vi "Set State.vi"(0 "Controller in":refnum<class "Controller.lvclass">, 1 "State":bool, 5 "error in":errorcluster) -> (14 "Controller out":refnum<class "Controller.lvclass">, 19 "error out":errorcluster)   [LabVIEW 2014, in "Controller.lvlib" / "Change Filter State.lvclass"]
uses:
  Change Filter State.lvclass
  Controller.lvclass
  SuperActor/Ex Nested.lvclass/Ex Nested.ctl
  Controller.lvclass/Controller.ctl
  <vilib>/DAQmx/write.llb/DAQmx Write (Digital 1D Bool NChan 1Samp 1Line).vi
  SuperActor/Read CVT Session.vi
  SuperActor/Read Log Session.vi
  Accessors/Read Filter Task.vi
  Accessors/Read Switch DVR.vi
  <vilib>/DAQmx/miscellaneous.llb/DAQmx Fill In Error Info.vi
  <userlib>/_Session Fwk/Session - Root.lvclass
  reusable/Switch/Switch.lvclass
  reusable/Session APIs/Session Log/System Log.lvclass
  reusable/Session APIs/CVT/CVT.lvclass
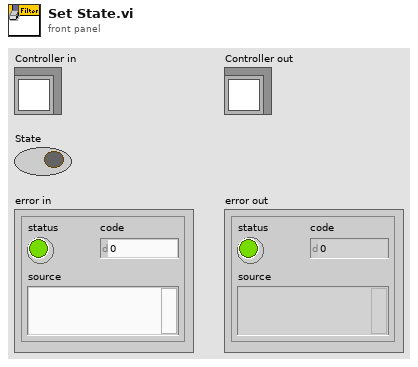
[diagram p1: front panel]
types:
  T1 = typedef "Session - Root.lvclass/Session Handle.ctl" = refnum<data-value>
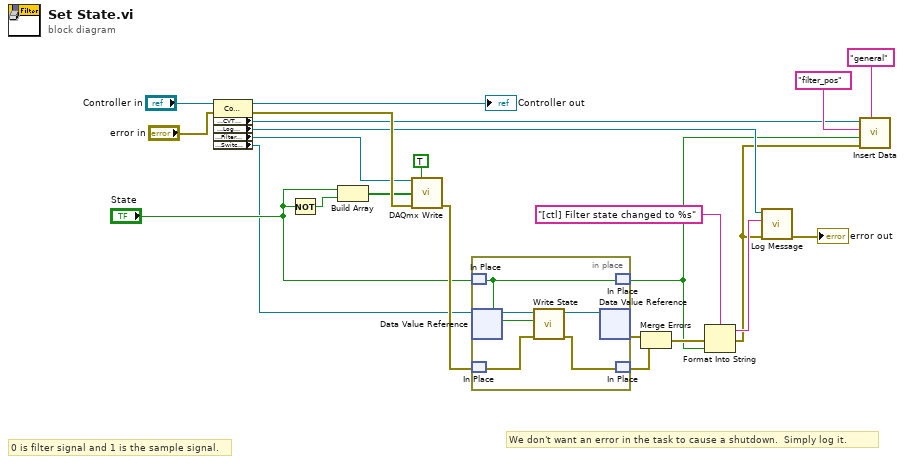
[diagram p0: block diagram]
diagram:
  # "0 is filter signal and 1 is the sample signal."
  # "We don't want an error in the task to cause a shutdown.  Simply log it."
  n1 = property class="Controller"(reference="Controller in", error in="error in") -> (reference out=→"Controller out":refnum<class "Controller.lvclass">, error out=w17:errorcluster, "Accessors:CVT Session"=w10:T1, "Accessors:Log Session"=w11:T1, "Accessors:Filter Task"=w1:refnum<k21>, "Accessors:Switch DVR"=w2:refnum<data-value>)
  n2 = Not(x="State") -> (.not. x?=w16:bool)
  n3 = Build Array("State", w16) -> (w15:bool[])
  n4 = call-poly <vilib>:"DAQmx Write.vi"("task/channels in"=w1, "auto start"=TRUE, "data"=w15, "error in"=w17) -> ("error out"=w8:errorcluster)  [unwired: 9 in, 2 out]
  n5 = in-place {
    n6 = in-place-match #1("State") -> (w24:bool)
    n7 = in-place-dvr #2(w2) -> (w28:refnum<class "Switch.lvclass">)  [unwired: 1 out]
    n8 = in-place-match #3(w8) -> (w25:errorcluster)
    n9 = call-dynamic "Write State.vi"("error in"=w25, "State"=w24, "Switch in"=w28) -> ("error out"=w26:errorcluster, "Switch out"=w27:refnum<class "Switch.lvclass">)  [unwired: 7 in]
    n10 = in-place-dvr #2(w27) -> (w23:errorcluster)  [unwired: 1 out]
    n11 = in-place-match #1(w24) -> (w3:bool)
    n12 = in-place-match #3(w26) -> (w9:errorcluster)
  }
  n13 = Merge Errors(w23, w9) -> (w7:errorcluster)
  n14 = Format Into String(format string="[ctl] Filter state changed to %s" ("MSG In"), error in=w7, w3) -> (resulting string=w18:string, error out=w5:errorcluster)  [unwired: 1 in]
  n15 = call "Log Message.vi"("error in"=w5, "MSG In"=w18, "session in"=w11) -> ("error out"=→"error out":errorcluster)  [unwired: 7 in, 1 out]
  n16 = call "Insert Data.vi"("Group"="general", "error in"=w5, "Data"=w3, "tag"="filter_pos", "CVT Session In"=w10) -> ()  [unwired: 5 in, 2 out]
